vi "Serialize.vi"(8 "error in":errorcluster, 9 "OwningElement in":refnum<k20>, 10 "Document in":refnum<k20>, 11 "DateTimeMeasure in":refnum<class "DateTimeMeasure.lvclass">) -> (0 "error out":errorcluster, 1 "OwningElement out":refnum<k20>, 2 "Document out":refnum<k20>, 3 "DateTimeMeasure out":refnum<class "DateTimeMeasure.lvclass">)   [LabVIEW 2021, in "ProligentXMLGenerator.lvlib" / "DateTimeMeasure.lvclass"]
uses:
  DateTimeMeasure.lvclass
  DateTimeMeasure.lvclass/DateTimeMeasure.ctl
  Base/DOMSupport/DOMSupport.lvlib
  Measure/Measure.lvclass
  <vilib>/xml/NI_XML.lvlib
  <vilib>/xml/Close Reference(Node).vi
  MeasureLimit/MeasureLimit.lvclass
  Base/Attribute/Attribute.lvclass
  Base/DateTime/DateTime.lvclass
  C:/Projects/proligent-xml-generator-labview/src/ProligentXMLGenerator/Measure/Measure/Measure.lvclass
  Base/MeasureKind/MeasureKind.lvclass
  C:/Projects/proligent-xml-generator-labview/src/ProligentXMLGenerator/Base/Attribute/Attribute.lvclass
  C:/Projects/proligent-xml-generator-labview/src/ProligentXMLGenerator/Base/MeasureKind/MeasureKind.lvclass
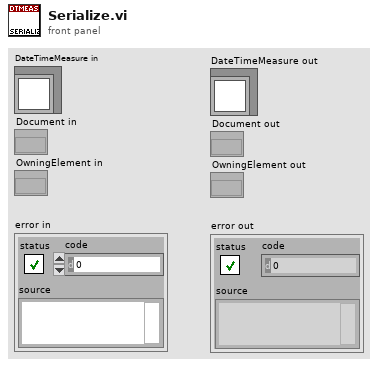
[diagram p1: front panel]
types:
  T1 = typedef "ProligentXMLGenerator.lvlib/DateTimeMeasure.lvclass/Data.ctl" = cluster{"Value":refnum<class "DateTime.lvclass">, "TimeZoneInfoId":string}
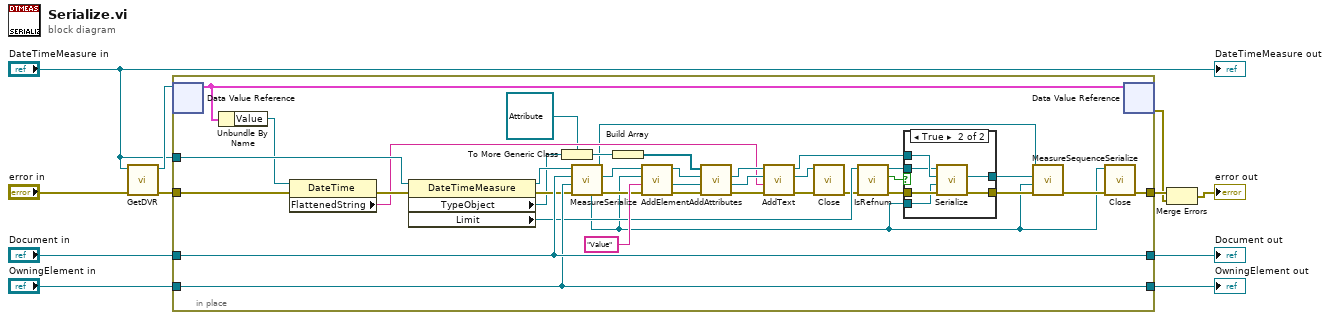
[diagram p0: block diagram]
diagram:
  n1 = call "GetDVR.vi"("error in"="error in", "DateTimeMeasure"="DateTimeMeasure in") -> ("error out"=w4:errorcluster, "DVRReference"=w3:refnum<data-value>)  [unwired: 8 in]
  n2 = in-place "In Place Element Structure" {
    in-place-border: [w38] -> w5
    in-place-border: "Document in" -> [w46]
    in-place-border: w4 -> [w45]
    in-place-border: "OwningElement in" -> [w44]
    in-place-border: [w44] -> w7
    in-place-border: [w46] -> w6
    in-place-border: "DateTimeMeasure in" -> [w41]
    n3 = in-place-dvr #1(w3) -> (w48:T1)  [unwired: 1 out]
    n4 = Unbundle By Name(w48) -> ("Value"=w21:refnum<class "DateTime.lvclass">)
    n5 = property on="Property Node" class="DateTime"(reference=w21, error in=w45) -> (error out=w22:errorcluster, "FlattenedString"=w20:string)  [unwired: 1 out]
    n6 = property on="Property Node" class="DateTimeMeasure"(reference=w41, error in=w22) -> (reference out=w33:refnum<class "DateTimeMeasure.lvclass">, error out=w42:errorcluster, "TypeObject"=w18:refnum<class "MeasureKind.lvclass">, "Limit"=w27:refnum<class "MeasureLimit.lvclass">)
    n7 = To More Generic Class(target class=refnum<class "Attribute.lvclass"> refnum ("ProligentResultProcessor:Attribute"), reference=w18) -> (generic class reference=w19:refnum<class "Attribute.lvclass">)
    n8 = call "MeasureSerialize.vi"("error in"=w42, "OwningElement in"=w44, "Document in"=w46, "Measure in"=w33) -> ("error out"=w31:errorcluster, "Document out"=w32:refnum<k20>, "Measure in"=w14:refnum<class "DateTimeMeasure.lvclass">, "Element"=w13:refnum<k20>)  [unwired: 3 in, 1 out]
    n9 = Build Array(w19) -> (w47:refnum<class "Attribute.lvclass">[])
    n10 = call "AddElement.vi"("error in"=w31, "Name"="Value", "OwningElement in"=w13, "Document in"=w32) -> ("error out"=w37:errorcluster, "NewElement"=w39:refnum<k20>, "Document out"=w40:refnum<k20>)  [unwired: 4 in, 1 out]
    n11 = call "AddAttributes.vi"("error in"=w37, "OwningElement in"=w39, "Document in"=w40, "Attributes"=w47) -> ("error out"=w36:errorcluster, "OwningElement out"=w34:refnum<k20>, "Document out"=w35:refnum<k20>)  [unwired: 5 in]
    n12 = call "AddText.vi"("error in"=w36, "Text"=w20, "OwningElement in"=w34, "Document in"=w35) -> ("error out"=w24:errorcluster, "OwningElement out"=w25:refnum<k20>, "Document out"=w26:refnum<k20>)  [unwired: 5 in]
    n13 = call-poly <vilib>:"Close.vi"("error in (no error)"=w24, "node"=w25) -> ("error out"=w23:errorcluster)  [unwired: 7 in]
    n14 = call "IsRefnum.vi"("error in"=w23, "MeasureLimit in"=w27) -> ("error out"=w30:errorcluster, "IsRefnum"=w29:bool, "MeasureLimit out"=w28:refnum<class "MeasureLimit.lvclass">)  [unwired: 7 in]
    n15 = case shown="True" w29 {
      tunnel: w30 -> [w50 w54]
      tunnel: [w50 w56] -> w16
      tunnel: w28 -> [_ w53]
      tunnel: w26 -> [w49 w55]
      tunnel: w13 -> [_ w52]
      tunnel: [w49 w51] -> w12
      frame False {
      }
      frame True {
        n16 = call "Serialize.vi"("error in"=w54, "OwningElement in"=w52, "Document in"=w55, "MeasureLimit in"=w53) -> ("error out"=w56:errorcluster, "Document out"=w51:refnum<k20>)  [unwired: 4 in, 2 out]
      }
    }
    n17 = call "MeasureSequenceSerialize.vi"("error in"=w16, "OwningElement in"=w13, "Document in"=w12, "Measure in"=w14) -> ("error out"=w15:errorcluster)  [unwired: 4 in, 3 out]
    n18 = call-poly <vilib>:"Close.vi"("error in (no error)"=w15, "node"=w13) -> ("error out"=w38:errorcluster)  [unwired: 7 in]
    n19 = in-place-dvr #1(w48) -> (w2:errorcluster)  [unwired: 1 out]
  }
  "Document out" <- w6
  "OwningElement out" <- w7
  n20 = Merge Errors(w5, w2) -> (→"error out":errorcluster)
  "DateTimeMeasure out" <- "DateTimeMeasure in"
